vi "Cull and Group.vi"(8 "Min Compnt %":dbl=15.0, 9 "Score Cutoff %":dbl=70.0, 10 "Sorted Data":dbl[][](array[numeric])) -> (2 "Best Targets above cutoff":T1(array[cluster]))   [LabVIEW 2025]
doc: "Examine the particle measurements to find the most likely pair that make up the target. This primarily compares the edges of the bounding boxes. It then returns information about the best two targets, notably the rectangle sourrounding the particles and the score."
panel:
  out "Grouping Scores":T2(array[cluster])
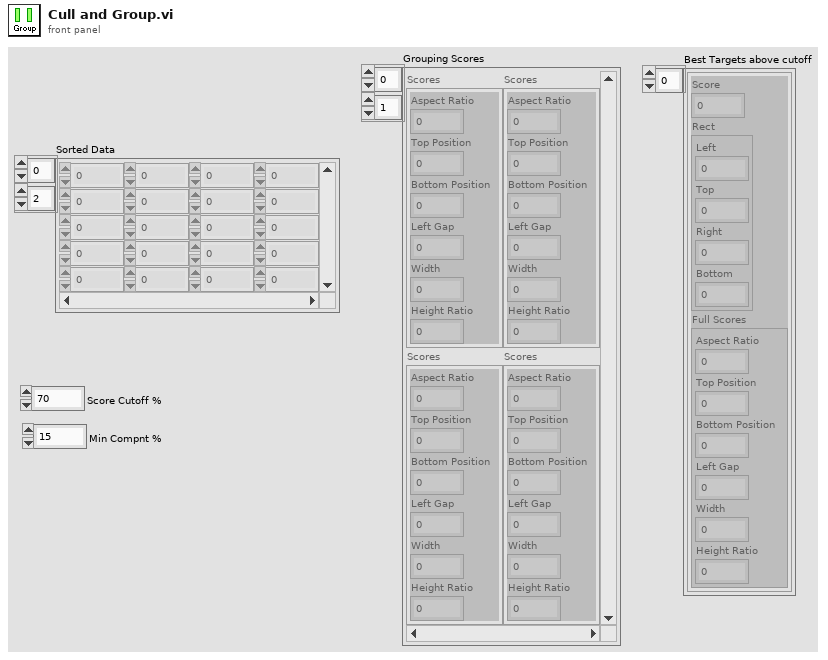
[diagram p1: front panel]
types:
  T1 = cluster{"Score":dbl, "Rect":cluster{"Left":dbl, "Top":dbl, "Right":dbl, "Bottom":dbl}, "Full Scores":cluster{"Aspect Ratio":dbl, "Top Position":dbl, "Bottom Position":dbl, "Left Gap":dbl, "Width":dbl, "Height Ratio":dbl}}[]
  T2 = cluster{"Aspect Ratio":dbl, "Top Position":dbl, "Bottom Position":dbl, "Left Gap":dbl, "Width":dbl, "Height Ratio":dbl}[][]
  T3 = cluster{"Left":dbl, "Top":dbl, "Right":dbl, "Bottom":dbl}
  T4 = cluster{"Aspect Ratio":dbl, "Strip Width":dbl, "Bottom Position":dbl, "Left Gap":dbl, "Width":dbl, "Height Ratio":dbl}
  T5 = cluster{dbl, "Rect":cluster{"Left":dbl, "Top":dbl, "Right":dbl, "Bottom":dbl}, "Scores":cluster{"Aspect Ratio":dbl, "Strip Width":dbl, "Bottom Position":dbl, "Left Gap":dbl, "Width":dbl, "Height Ratio":dbl}}
  T6 = cluster{dbl, "Rect":cluster{"Left":dbl, "Top":dbl, "Right":dbl, "Bottom":dbl}, "Scores":cluster{"Aspect Ratio":dbl, "Strip Width":dbl, "Bottom Position":dbl, "Left Gap":dbl, "Width":dbl, "Height Ratio":dbl}}[]
  T7 = cluster{"Aspect Ratio":bool, "Strip Width":bool, "Bottom Position":bool, "Left Gap":bool, "Width":bool, "Height Ratio":bool}
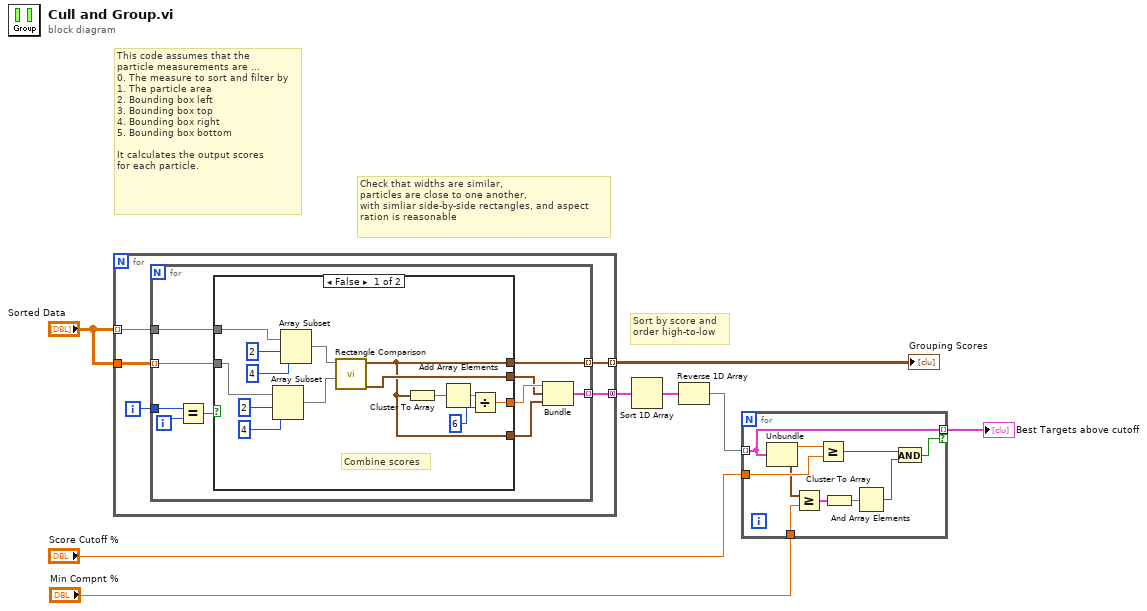
[diagram p0: block diagram]
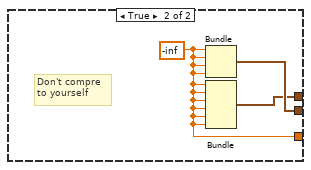
[diagram p2: hidden frame]
diagram:
  # "Sort by score and\norder high-to-low"
  # "Check that widths are similar,\nparticles are close to one another,\nwith simliar side-by-side rectangles, and aspect\nration is reasonable"
  # "This code assumes that the\nparticle measurements are ...\n0. The measure to sort and filter by\n1. The particle area\n2. Bounding box left\n3. Bounding box top\n4. Bounding box right\n5. Bounding box bottom\n\nIt calculates the output scores\nfor each particle."
  n1 = for {
    tunnel: "Sorted Data" -> [w13] mode=indexing
    tunnel: "Sorted Data" -> [w12]
    tunnel: [w11] -> w8 mode=indexing
    tunnel: [w9] -> w6 mode=concatenating
    i -> [w10]
    n2 = for {
      tunnel: w13 -> [w23]
      tunnel: w12 -> [w21] mode=indexing
      tunnel: [w20] -> w11 mode=indexing
      tunnel: w10 -> [w19]
      tunnel: [w15] -> w9 mode=indexing
      i -> [w18]
      n3 = Equal?(x=w19, y=w18) -> (x = y?=w22:bool)
      n4 = case shown="False" w22 {
        tunnel: w23 -> [w35 _]
        tunnel: w21 -> [w32 _]
        tunnel: [w24 w39] -> w20
        tunnel: [w25 w38] -> w17
        tunnel: [w28 w40] -> w16
        tunnel: [w24 _] -> w14
        frame False {
          # "Combine scores"
          n5 = Array Subset(array=w32, index=2, length=4) -> (w29:dbl[])
          n6 = Array Subset(array=w35, index=2, length=4) -> (w30:dbl[])
          n7 = call "Rectangle Comparison.vi"("Second"=w29, "First"=w30) -> ("Rect"=w28:T3, "Scores"=w24:T4)  [unwired: 8 in]
          n8 = Cluster To Array(cluster=w24) -> (array=w31:dbl[])
          n9 = Add Array Elements(numeric array=w31) -> (sum=w26:dbl)
          n10 = Divide(x=w26, y=6 ("length")) -> (x/y=w25:dbl)
        }
        frame True {
          w38 = -inf
          # "Don't compre\nto yourself"
          n11 = Bundle(w38, w38, w38, w38) -> (w40:cluster{dbl, dbl, dbl, dbl})  [unwired: 1 in]
          n12 = Bundle(w38, w38, w38, w38, w38, w38) -> (w39:cluster{dbl, dbl, dbl, dbl, dbl, dbl})  [unwired: 1 in]
        }
      }
      n13 = Bundle(w17, "Rect"=w16, "Scores"=w14) -> (w15:T5)  [unwired: 1 in]
    }
  }
  "Grouping Scores" <- w8
  n14 = Sort 1D Array(array=w6) -> (sorted array=w5:T6)
  n15 = Reverse 1D Array(array=w5) -> (reversed array=w4:T6)
  n16 = for {
    tunnel: w4 -> [w50] mode=indexing
    tunnel: [w50] -> w2 mode=indexing if=w41
    tunnel: "Score Cutoff %" -> [w48]
    tunnel: "Min Compnt %" -> [w46]
    n17 = Unbundle(w50) -> (w49:dbl, "Scores"=w47:T4)  [unwired: 1 out]
    n18 = Greater Or Equal?(x=w47, y=w46) -> (x >= y?=w45:T7)
    n19 = Greater Or Equal?(x=w49, y=w48) -> (x >= y?=w42:bool)
    n20 = Cluster To Array(cluster=w45) -> (array=w44:bool[])
    n21 = And Array Elements(Boolean array=w44) -> (logical AND=w43:bool)
    n22 = And(x=w42, y=w43) -> (x .and. y?=w41:bool)
  }
  "Best Targets above cutoff" <- w2
